vi "TWM Client Close.vi"(7 "end of packet key":string="TWM:command:EndOfPacket", 8 "error in":errorcluster, 11 "handle in":i32) -> (0 "error out":errorcluster)   [LabVIEW 2020, in "TWM Client.lvlib"]
doc: "Closes pipe to the TWM server. Will be executed even if error is at input."
uses:
  TWM Client.lvlib
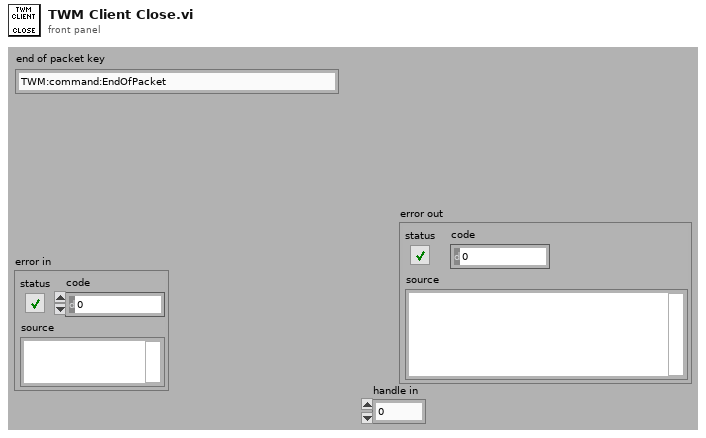
[diagram p1: front panel]
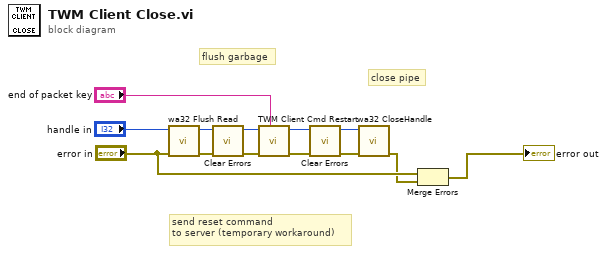
[diagram p0: block diagram]
diagram:
  # "close pipe"
  # "send reset command\nto server (temporary workaround)"
  # "flush garbage"
  n1 = call "wa32 Flush Read.vi"("error in"="error in", "handle"="handle in") -> ("error out"=w6:errorcluster, "handle out"=w7:i32)  [unwired: 7 in, 1 out]
  n2 = call <vilib>:"Clear Errors.vi"("error in (no error)"=w6) -> ("error out"=w5:errorcluster)  [unwired: 5 in, 1 out]
  n3 = call "TWM Client Cmd Restart.vi"("end of packet key"="end of packet key", "error in"=w5, "handle"=w7) -> ("error out"=w4:errorcluster, "handle out"=w2:i32)  [unwired: 7 in]
  n4 = call <vilib>:"Clear Errors.vi"("error in (no error)"=w4) -> ("error out"=w3:errorcluster)  [unwired: 5 in, 1 out]
  n5 = call "wa32 CloseHandle.vi"("error in"=w3, "handle"=w2) -> ("error out"=w1:errorcluster)  [unwired: 9 in]
  n6 = Merge Errors("error in", w1) -> (→"error out":errorcluster)
